vi "Get Motor Stall Percentage.vi"(9 "Observed Encoder Rate":dbl, 10 "PWM Output":dbl) -> (1 "Percent Of Potential Speed":dbl, 2 "Maximum Potential Speed":dbl)   [LabVIEW 2012]
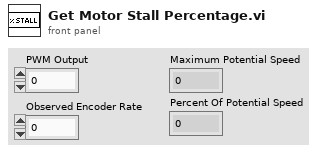
[diagram p1: front panel]
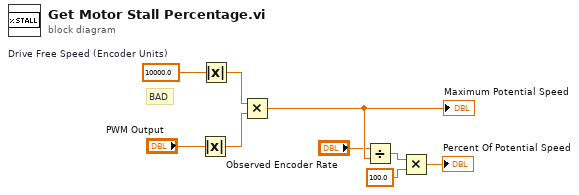
[diagram p0: block diagram]
diagram:
  w9 = 10000.0  # Drive Free Speed (Encoder Units)
  # "BAD"
  n1 = Absolute Value(x="PWM Output") -> (abs(x)=w6:dbl)
  n2 = Absolute Value(x=w9) -> (abs(x)=w7:dbl)
  n3 = Multiply(x=w7, y=w6) -> (x*y=w5:dbl)
  "Maximum Potential Speed" <- w5
  n4 = Divide(x="Observed Encoder Rate", y=w5) -> (x/y=w3:dbl)
  n5 = Multiply(x=w3, y=100.0) -> (x*y=→"Percent Of Potential Speed":dbl)
